vi "SVPO Integration (1 CH DBL Array).vi"(6 "reset filters":bool, 9 "highpass cutoff frequency [Hz]":dbl=1.0 format="%.2f", 10 "sampling rate [Hz]":dbl=1.0, 11 "scaled signal [EU]":dbl[](array[numeric])) -> (3 "integrated signal [EU*s]":dbl[](array[numeric]))   [LabVIEW 2017, in "SoundVib_Integration.lvlib"]
doc: "Converts acceleration to velocity or velocity to displacement using a time-domain waveform as the input. Wire data to the <B>scaled signal [EU]</B> input to determine the polymorphic instance to use or manually select the instance. This VI performs Single Integration only. You can pass the integrated signal [EU*s] output to the scaled signal [EU] input of second call to this VI to perform double integration."
uses:
  <vilib>/addons/Sound and Vibration/svt_Integration/SoundVib_Integration.lvlib
  <vilib>/addons/Sound and Vibration/svt_Integration/subVIs/svl_Apply Highpass Filter with IC.vi
  <vilib>/addons/Sound and Vibration/svt_Integration/subVIs/svl_Low Pass [Order 1] No State.vi
  <vilib>/addons/Sound and Vibration/svt_Integration/subVIs/svl_Design HighPass Filter.vi
  <vilib>/addons/Sound and Vibration/svt_Integration/subVIs/svl_RC Filter Coefficients.vi
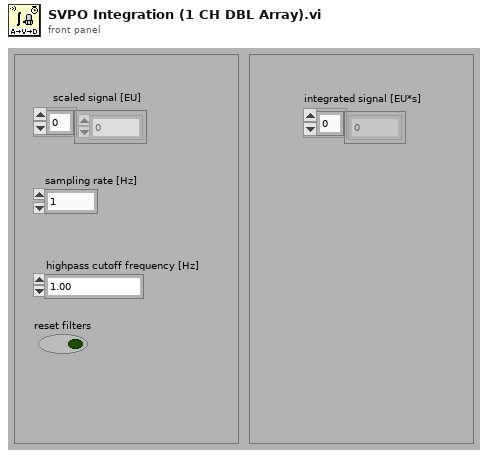
[diagram p1: front panel]
types:
  T1 = typedef "svc_Integration State.ctl" = cluster{"filter coefficents":cluster{"integration filter coefficients":cluster{"beta":dbl, "gamma":dbl, "alpha":dbl}, "highpass filter coefficients":cluster{"filter structure":enum32{"IIR 2nd Order", "IIR 4th Order"}, "Reverse Coefficients":dbl[], "Forward Coefficients":dbl[]}}, "filter state":cluster{"initial integration fiter state":cluster{"x(n-1) state":dbl, "y(n-1) state":dbl, "x(n-2) state":dbl, "y(n-2) state":dbl}, "initial highpass filter state":dbl[]}}
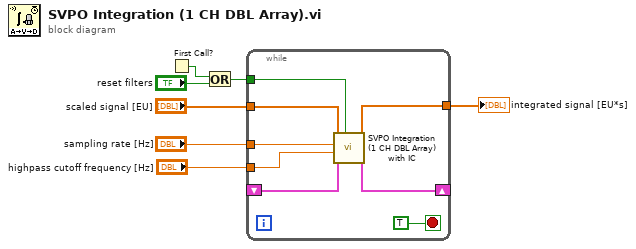
[diagram p0: block diagram]
diagram:
  n1 = First Call?() -> (First Call?: T/F=w7:bool)
  n2 = Or(x=w7, y="reset filters") -> (x .or. y?=w5:bool)
  n3 = while {
    tunnel: w5 -> [w8]
    tunnel: "scaled signal [EU]" -> [w15]
    tunnel: "sampling rate [Hz]" -> [w14]
    tunnel: "highpass cutoff frequency [Hz]" -> [w13]
    tunnel: [w12] -> w1
    shift-right: [w11] -> _
    shift-left: _ -> [w10]
    stop <- TRUE stop-if-true
    n4 = call <vilib>:"SVPO Integration (1 CH DBL Array) with IC.vi"("reset filters"=w8, "initial conditions"=w10, "highpass cutoff frequency [Hz]"=w13, "sampling rate [Hz]"=w14, "scaled signal [EU]"=w15) -> ("final conditions"=w11:T1, "integrated signal [EU*s]"=w12:dbl[])  [unwired: 5 in]
  }
  "integrated signal [EU*s]" <- w1
